vi "Open Help File.vi"() -> ()   [LabVIEW 2021]
uses:
  <vilib>/NI VeriStand/Custom Device API/Custom Device API.lvlib
  NationalInstruments.VeriStand.SystemStorage
  <vilib>/NI VeriStand/Custom Device API/Custom Device Item Ref.ctl
panel:
  in  "Node Ptr":T1 format="%.0x"
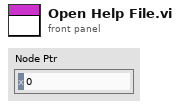
[diagram p1: front panel]
types:
  T1 = typedef "Custom Device API.lvlib/Custom Device Item Ref.ctl" = u64
  T2 = typedef "Custom Device API.lvlib/Custom Device Pointer.ctl" = refnum<k24>
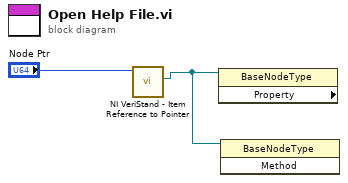
[diagram p0: block diagram]
diagram:
  n1 = call <vilib>:"NI VeriStand - Item Reference to Pointer.vi"("Item Ref in"="Node Ptr") -> ("Node Pointer"=w1:T2)  [unwired: 7 in, 3 out]
  n2 = property class="BaseNodeType" props=[](reference=w1) -> ()  [unwired: 1 in, 3 out]
  n3 = invoke class="BaseNodeType" method=#-1(reference=w1) -> ()  [unwired: 2 in, 3 out]
